vi "unflattenFromString.vi"(8 "error in (no error)":errorcluster, 10 "binary string":string, 11 "Task Status in":refnum<class "Task Status.lvclass">) -> (0 "error out":errorcluster, 3 "Task Status out":refnum<class "Task Status.lvclass">)   [LabVIEW 2017, in "Message Interface.lvlib" / "Task Status.lvclass"]
uses:
  Task Status.lvclass
  C:/Users/Public/Documents/wc/BuildFarm/src/LabVIEW/vi.lib/BenjaminR/Build Farm/Classes/Message Interface/Status/Status.lvclass
  Status/Status.lvclass/Status.ctl
  Status/Read Item Name.vi
  Status/Write Item Name.vi
  Status/Status.lvclass
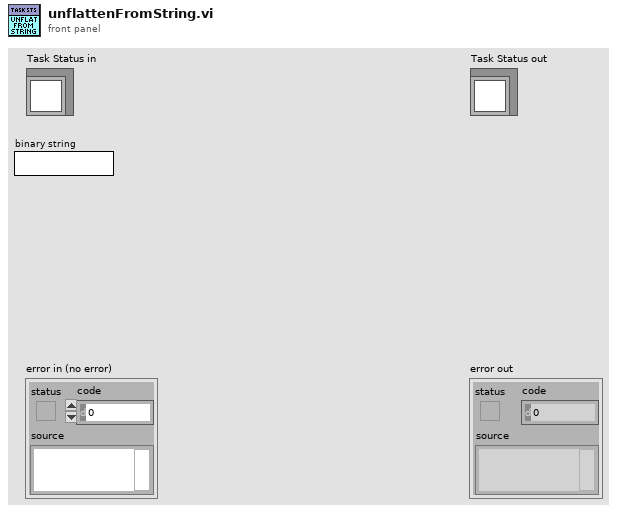
[diagram p1: front panel]
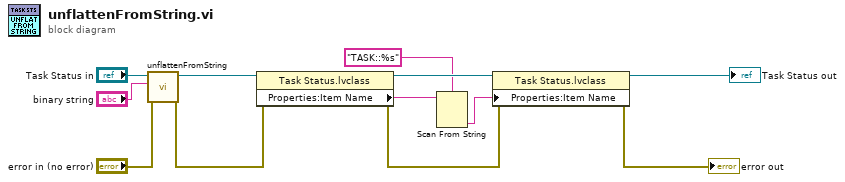
[diagram p0: block diagram]
diagram:
  n1 = call-parent "unflattenFromString.vi"("error in (no error)"="error in (no error)", "binary string"="binary string", "iMessage in"="Task Status in") -> ("error out"=w4:errorcluster, "iMessage out"=w5:refnum<class "Task Status.lvclass">)  [unwired: 7 in]
  n2 = property class="Task Status.lvclass"(reference=w5, error in=w4) -> (reference out=w9:refnum<class "Task Status.lvclass">, error out=w1:errorcluster, "Properties:Item Name"=w8:string)
  n3 = Scan From String(format string="TASK::%s" ("string"), input string=w8) -> (output 1=w6:string)  [unwired: 3 in, 3 out]
  n4 = property class="Task Status.lvclass"(reference=w9, error in=w1, "Properties:Item Name"=w6) -> (reference out=→"Task Status out":refnum<class "Task Status.lvclass">, error out=→"error out":errorcluster)
